vi "Set Scan Parameters.vi"(8 "error in (no error)":errorcluster, 11 "Abstract Delay Line in":refnum<class "Abstract Delay Line.lvclass">) -> (0 "error out":errorcluster, 3 "Abstract Delay Line out":refnum<class "Abstract Delay Line.lvclass">)   [LabVIEW 2016, in "Delay Line.lvlib" / "Abstract Delay Line.lvclass"]
uses:
  Abstract Delay Line.lvclass
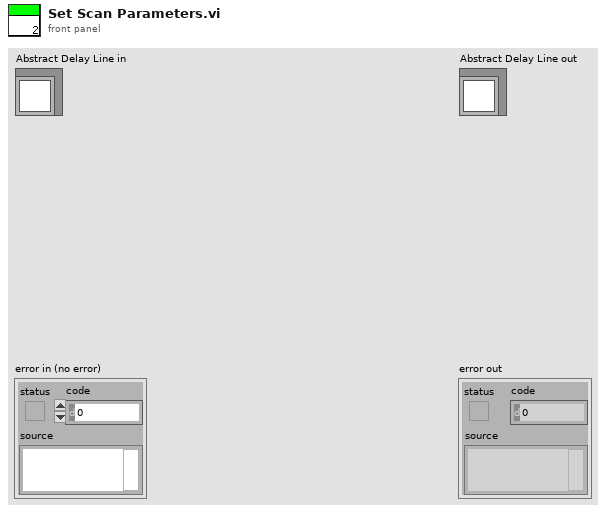
[diagram p1: front panel]
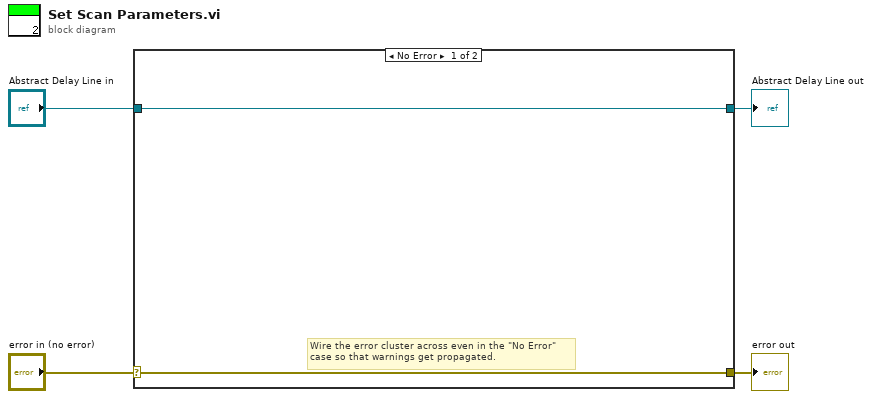
[diagram p0: block diagram]
diagram:
  n1 = case shown="No Error" "error in (no error)" {
    selector: "error in (no error)" -> [w5 w8]
    tunnel: [w5 w8] -> w3
    tunnel: [w6 w7] -> w1
    tunnel: "Abstract Delay Line in" -> [w6 w7]
    frame No Error {
      # "Wire the error cluster across even in the \"No Error\"\ncase so that warnings get propagated."
    }
    frame Error {
    }
  }
  "error out" <- w3
  "Abstract Delay Line out" <- w1
